vi "PAN_ProcCmd.vi"(0 "Translations":refnum<vi>, 1 "modpath":path, 4 "addid":refnum<vi>, 5 "Modules":refnum<vi>, 6 "cinfo":string, 7 "command in":string, 9 "exp time":dbl, 11 "shutdown":refnum<vi>, 12 "cmdQ":refnum<queue>, 13 "internal queue in":refnum<queue>, 14 "nodeID":string) -> (2 "init timeout":i32, 3 "DHE_DBSRef":T2, 8 "response":string, 10 "exp time out":dbl, 15 "shutdown":bool)   [LabVIEW 2016]
uses:
  Modules/DBSHAND/private/vis/DatabaseHand_RefNum.ctl
  PAN_actionsSTruct.ctl
  PAN_cmdStruct.ctl
panel:
  in  "action struct 2":T1
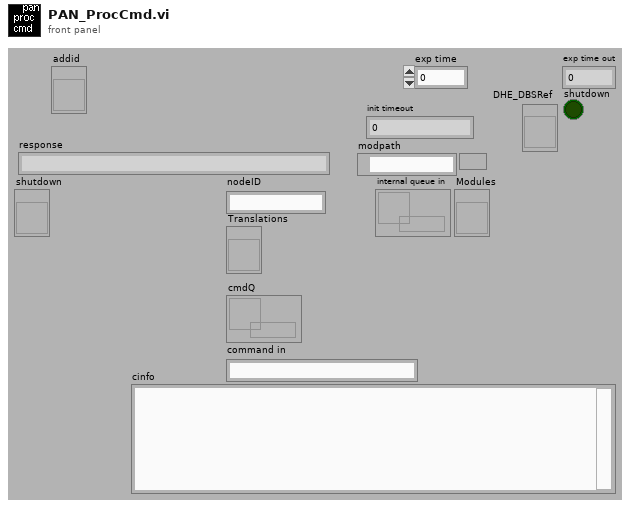
[diagram p1: front panel]
types:
  T1 = typedef "PAN_actionsSTruct.ctl" = cluster{"command":string, "timeout":u32}
  T2 = typedef "DatabaseHand_RefNum.ctl" = refnum<vi>
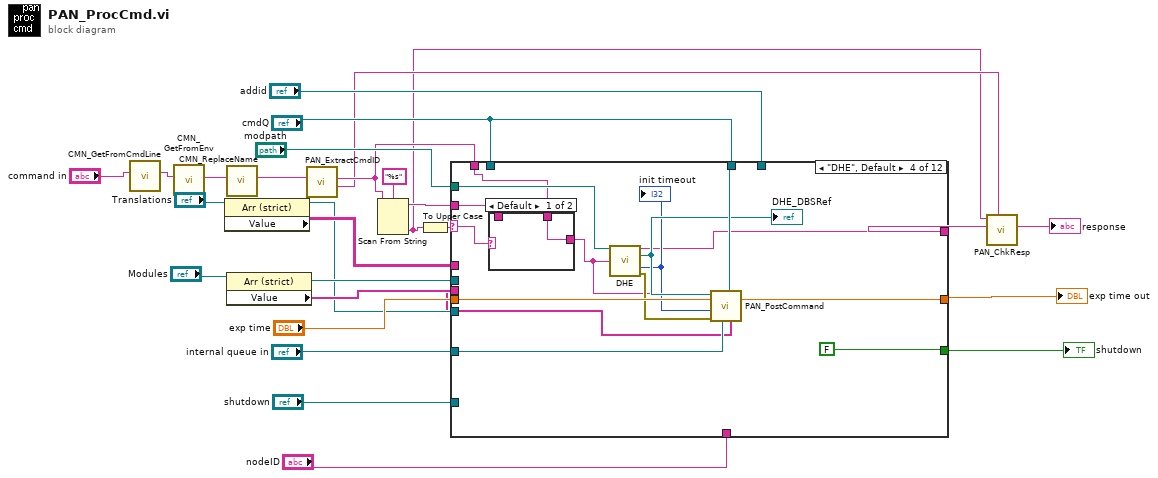
[diagram p0: block diagram]
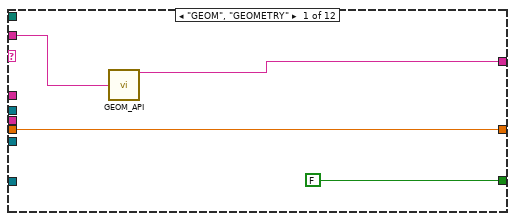
[diagram p2: hidden frame]
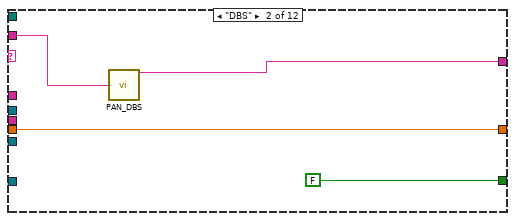
[diagram p3: hidden frame]
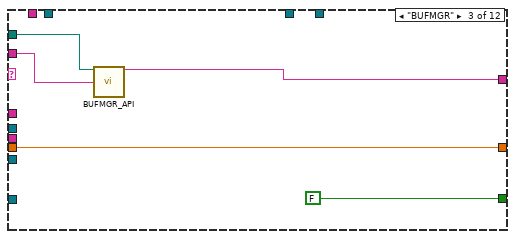
[diagram p4: hidden frame]
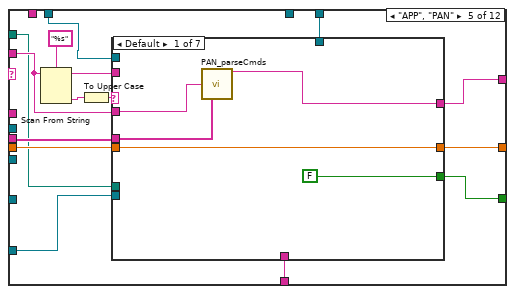
[diagram p6: hidden frame]
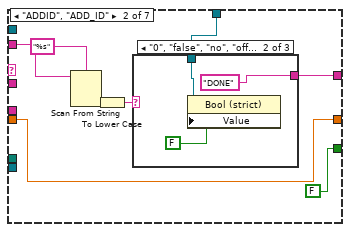
[diagram p7: hidden frame]
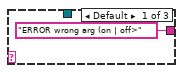
[diagram p8: hidden frame]
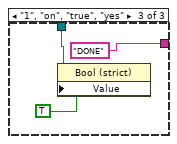
[diagram p9: hidden frame]
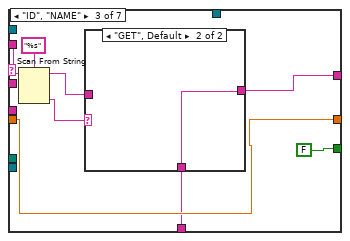
[diagram p10: hidden frame]
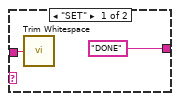
[diagram p11: hidden frame]
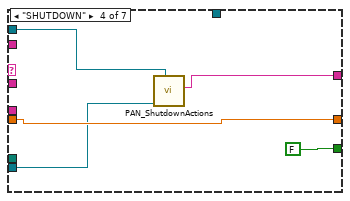
[diagram p12: hidden frame]
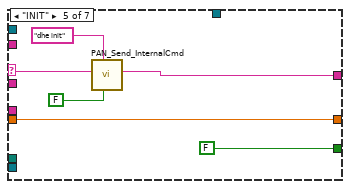
[diagram p13: hidden frame]
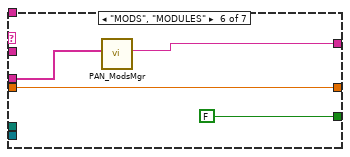
[diagram p14: hidden frame]
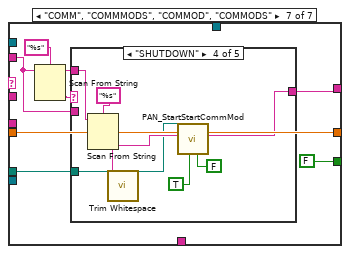
[diagram p15: hidden frame]
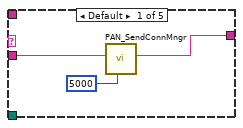
[diagram p16: hidden frame]
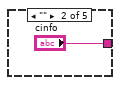
[diagram p17: hidden frame]
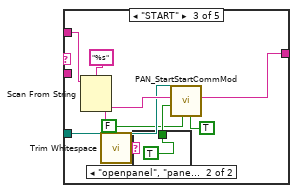
[diagram p18: hidden frame]
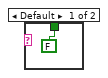
[diagram p19: hidden frame]
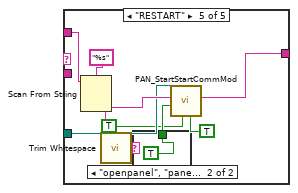
[diagram p20: hidden frame]
diagram:
  n1 = call "CMN_GetFromCmdLine.vi"("str in"="command in") -> ("str out"=w7:string)  [unwired: 10 out]
  n2 = call "CMN_GetFromEnv.vi"("str in"=w7) -> ("str out"=w5:string)  [unwired: 10 out]
  n3 = property class="Arr (strict)"(reference="Translations") -> (reference out=w12:refnum<vi>, "Value"=w13:string[][])  [unwired: 1 in, 1 out]
  n4 = call "CMN_ReplaceName.vi"("name in"=w5) -> ("name out"=w4:string)  [unwired: 1 in, 9 out]
  n5 = property class="Arr (strict)"(reference="Modules") -> (reference out=w15:refnum<vi>, "Value"=w16:string[])  [unwired: 1 in, 1 out]
  n6 = call "PAN_ExtractCmdID.vi"("command in"=w4) -> ("cmdID"=w2:string, "cmd out"=w3:string)  [unwired: 9 out]
  n7 = Scan From String(format string="%s", input string=w3) -> (remaining string=w25:string, output 1=w1:string)  [unwired: 2 in, 3 out]
  n8 = To Upper Case(1:w1) -> (0:w26:string)
  n9 = case shown="\"DHE\", Default" w26 {
    selector: w26 -> [_ _ _ w44 _ _ _ _ _ _ _ _]
    tunnel: w3 -> [_ _ _ w41 _ _ _ _ _ _ _ _]
    tunnel: [w31 w35 w40 w46 w68 w166 w171 w181 "DONE" ("ImmedReplyString") "DONE" ("ImmedReplyString") w211 "" ("ImmedReplyString")] -> w23
    tunnel: w25 -> [w29 w33 w38 w47 w63 w164 w169 w173 w195 _ _ _]
    tunnel: "exp time" -> [w30 w34 w39 w55 w65 w167 w172 w182 _ _ w212 _]
    tunnel: [w30 w34 w39 w54 w64 w167 w172 w182 0.0 ("exp time") 0.0 ("exp time") w212 0.0 ("exp time")] -> w24
    tunnel: "internal queue in" -> [_ _ _ w53 _ _ _ _ w198 _ _ _]
    tunnel: "cmdQ" -> [_ _ _ _ w67 _ _ _ _ w206 _ _]
    tunnel: "cmdQ" -> [_ _ _ w52 _ _ _ _ _ _ w210 _]
    tunnel: "modpath" -> [_ _ w37 w45 w58 _ _ w177 _ _ _ _]
    tunnel: w16 -> [_ _ _ w48 w66 _ _ w179 _ w203 _ _]
    tunnel: w13 -> [_ _ _ _ _ _ _ w180 _ _ _ _]
    tunnel: w15 -> [_ _ _ _ _ _ _ w176 _ _ _ _]
    tunnel: w12 -> [_ _ _ _ _ _ _ w175 _ _ _ _]
    tunnel: [FALSE FALSE FALSE FALSE w62 FALSE FALSE FALSE FALSE FALSE FALSE TRUE] -> w11
    tunnel: "nodeID" -> [_ _ _ _ w61 _ _ _ _ _ _ _]
    tunnel: "addid" -> [_ _ _ _ w60 _ _ _ _ _ _ _]
    tunnel: "shutdown" -> [_ _ _ _ w59 _ _ _ _ _ w209 _]
    frame "GEOM", "GEOMETRY" {
      n10 = call "GEOM_API.vi"("Cmd"=w29) -> ("ImmedReplyString"=w31:string)  [unwired: 1 in, 13 out]
    }
    frame "DBS" {
      n11 = call "PAN_DBS.vi"("Cmd"=w33) -> ("ImmedReplyString"=w35:string)  [unwired: 1 in, 13 out]
    }
    frame "BUFMGR" {
      n12 = call "BUFMGR_API.vi"("modpath"=w37, "Cmd"=w38) -> ("ImmedReplyString"=w40:string)  [unwired: 1 in, 12 out]
    }
    frame "DHE", Default {
      n13 = case shown="Default" w44 {
        tunnel: w41 -> [w56 _]
        tunnel: w47 -> [_ w57]
        tunnel: [w56 w57] -> w42
        frame Default {
        }
        frame "DHE" {
        }
      }
      n14 = call "DHE.vi"("modpath"=w45, "Cmd"=w42) -> ("ImmedReplyString"=w46:string, "DHE_DBSRef"=w51:T2, "TimeOut out"=w49:i32, "error out"=w50:errorcluster)  [unwired: 1 in, 9 out]
      "DHE_DBSRef" <- w51
      "init timeout" <- w49
      n15 = call "PAN_PostCommand.vi"("Modules"=w48, "cmdQ"=w52, "queue out"=w53, "command"=w42, "error in (no error)"=w50, "timeout"=w49, "orig exptime"=w55, "DHE_DBSRef"=w51) -> ("exp time"=w54:dbl)  [unwired: 3 out]
    }
    frame "APP", "PAN" {
      n16 = Scan From String(format string="%s", input string=w63) -> (remaining string=w69:string, output 1=w71:string)  [unwired: 2 in, 3 out]
      n17 = To Upper Case(1:w71) -> (0:w70:string)
      n18 = case shown="Default" w70 {
        selector: w70 -> [_ _ _ _ w112 _ _]
        tunnel: w69 -> [_ w85 w97 _ _ _ w121]
        tunnel: [w75 w78 w99 w106 w110 w117 w124] -> w68
        tunnel: [FALSE FALSE FALSE FALSE FALSE FALSE FALSE] -> w62
        tunnel: w67 -> [_ _ _ w105 _ _ _]
        tunnel: w66 -> [w73 _ _ _ _ w118 _]
        tunnel: w65 -> [w76 w80 w98 w107 w113 w116 w125]
        tunnel: [w76 w80 w98 w107 w113 w116 w125] -> w64
        tunnel: w63 -> [w74 _ _ _ _ _ _]
        tunnel: w61 -> [_ _ w93 _ _ _ _]
        tunnel: w60 -> [_ w79 _ _ _ _ _]
        tunnel: w59 -> [_ _ _ w104 _ _ _]
        tunnel: w58 -> [_ _ _ _ _ _ w119]
        frame Default {
          n19 = call "PAN_parseCmds.vi"("Cmd Option"=w74, "Modules"=w73) -> ("ImmedReplyString"=w75:string)  [unwired: 1 in, 12 out]
        }
        frame "ADDID", "ADD_ID" {
          n20 = Scan From String(format string="%s", input string=w85) -> (output 1=w82:string)  [unwired: 2 in, 4 out]
          n21 = To Lower Case(string=w82) -> (all lower case string=w81:string)
          n22 = case shown="\"0\", \"false\", \"no\", \"off\"" w81 {
            tunnel: w79 -> [_ w89 w92]
            tunnel: ["ERROR wrong arg (on | off>" ("response") "DONE" ("response") "DONE" ("response")] -> w78
            frame Default {
            }
            frame "0", "false", "no", "off" {
              n23 = property class="Bool (strict)"(reference=w89, "Value"=FALSE) -> ()  [unwired: 1 in, 2 out]
            }
            frame "1", "on", "true", "yes" {
              n24 = property class="Bool (strict)"(reference=w92, "Value"=TRUE) -> ()  [unwired: 1 in, 2 out]
            }
          }
        }
        frame "ID", "NAME" {
          n25 = Scan From String(format string="%s", input string=w97) -> (remaining string=w94:string, output 1=w95:string)  [unwired: 2 in, 3 out]
          n26 = case shown="\"GET\", Default" w95 {
            tunnel: ["DONE" ("ID") w103] -> w99
            tunnel: w94 -> [w101 _]
            tunnel: w93 -> [_ w103]
            frame "SET" {
              n27 = call <vilib>:"Trim Whitespace.vi"("string"=w101) -> ()  [unwired: 1 in, 1 out]
            }
            frame "GET", Default {
            }
          }
        }
        frame "SHUTDOWN" {
          n28 = call "PAN_ShutdownActions.vi"("cmdQ"=w105, "shutdownscr ref"=w104) -> ("response"=w106:string)  [unwired: 9 out]
        }
        frame "INIT" {
          n29 = call "PAN_Send_InternalCmd.vi"("wait response"=FALSE, "taskID"="dhe init", "command"=w112) -> ("response"=w110:string)  [unwired: 2 in, 6 out]
        }
        frame "MODS", "MODULES" {
          n30 = call "PAN_ModsMgr.vi"("Modules"=w118) -> ("response"=w117:string)  [unwired: 10 out]
        }
        frame "COMM", "COMMMODS", "COMMOD", "COMMODS" {
          n31 = Scan From String(format string="%s", input string=w121) -> (remaining string=w120:string, output 1=w122:string)  [unwired: 2 in, 3 out]
          n32 = case shown="\"SHUTDOWN\"" w122 {
            tunnel: [w127 "cinfo" w132 w144 w152] -> w124
            tunnel: w121 -> [w129 _ _ _ _]
            tunnel: w120 -> [_ _ w140 w150 w160]
            tunnel: w119 -> [_ _ w137 w147 w157]
            frame Default {
              n33 = call "PAN_SendConnMngr.vi"("timeout in ms (-1)"=5000, "command"=w129) -> ("resp"=w127:string)  [unwired: 1 in, 8 out]
            }
            frame "" {
            }
            frame "START" {
              n34 = Scan From String(format string="%s", input string=w140) -> (remaining string=w136:string, output 1=w138:string)  [unwired: 2 in, 3 out]
              n35 = call <vilib>:"Trim Whitespace.vi"("string"=w136) -> ("trimmed string"=w135:string)  [unwired: 1 in]
              n36 = case shown="\"openpanel\", \"panel\"" w135 {
                tunnel: [FALSE ("Front Panel Window:Open") TRUE ("Front Panel Window:Open")] -> w134
                frame Default {
                }
                frame "openpanel", "panel" {
                }
              }
              n37 = call "PAN_StartStartCommMod.vi"("start"=TRUE, "running"=FALSE, "ModPath"=w137, "openpanel"=w134, "commod"=w138) -> ("response"=w132:string)  [unwired: 1 in, 5 out]
            }
            frame "SHUTDOWN" {
              n38 = Scan From String(format string="%s", input string=w150) -> (remaining string=w146:string, output 1=w148:string)  [unwired: 2 in, 3 out]
              n39 = call <vilib>:"Trim Whitespace.vi"("string"=w146) -> ()  [unwired: 1 in, 1 out]
              n40 = call "PAN_StartStartCommMod.vi"("start"=FALSE, "running"=TRUE, "ModPath"=w147, "commod"=w148) -> ("response"=w144:string)  [unwired: 2 in, 5 out]
            }
            frame "RESTART" {
              n41 = Scan From String(format string="%s", input string=w160) -> (remaining string=w156:string, output 1=w158:string)  [unwired: 2 in, 3 out]
              n42 = call <vilib>:"Trim Whitespace.vi"("string"=w156) -> ("trimmed string"=w155:string)  [unwired: 1 in]
              n43 = case shown="\"openpanel\", \"panel\"" w155 {
                tunnel: [FALSE ("Front Panel Window:Open") TRUE ("Front Panel Window:Open")] -> w154
                frame Default {
                }
                frame "openpanel", "panel" {
                }
              }
              n44 = call "PAN_StartStartCommMod.vi"("start"=TRUE, "running"=TRUE, "ModPath"=w157, "openpanel"=w154, "commod"=w158) -> ("response"=w152:string)  [unwired: 1 in, 5 out]
            }
          }
        }
      }
    }
    frame "APPMACRO" {
      n45 = call "PAN_MacroCmd.vi"("timeout in ms (-1)"=-1, "Command"=w164) -> ("response"=w166:string)  [unwired: 1 in, 8 out]
    }
    frame "APPMACRONORESP" {
      n46 = call "PAN_MacroCmd.vi"("timeout in ms (-1)"=1, "Command"=w169) -> ("response"=w171:string)  [unwired: 1 in, 8 out]
    }
    frame "MOD" {
      n47 = call "PAN_ModCaller.vi"("CmdStringIn"=w173, "modpath"=w177) -> ("ImmedReplyString"=w181:string, "new mod"=w178:bool)  [unwired: 1 in, 11 out]
      n48 = case shown="True" w178 {
        tunnel: w180 -> [_ w190]
        tunnel: w179 -> [_ w189]
        tunnel: w173 -> [_ w188]
        tunnel: w177 -> [_ w187]
        tunnel: w176 -> [_ w186]
        tunnel: w175 -> [_ w184]
        frame False {
        }
        frame True {
          n49 = call "PAN_AddModule.vi"("Mods in"=w189, "Translations In"=w190, "modpath"=w187, "module name"=w188) -> ("Mods Out"=w185:string[], "Translations out"=w183:string[][])  [unwired: 6 out]
          n50 = property class="Arr (strict)"(reference=w186, "Value"=w185) -> ()  [unwired: 1 in, 2 out]
          n51 = property class="Arr (strict)"(reference=w184, "Value"=w183) -> ()  [unwired: 1 in, 2 out]
        }
      }
    }
    frame "BOOT" {
      n52 = Scan From String(format string="%d", input string=w195) -> (output 1=w193:i32)  [unwired: 2 in, 4 out]
      n53 = Bundle By Name(cluster="action struct 2", "command"="INIT", "timeout"=w193) -> (w200:T1)
      n54 = call "PAN_VAR_Status.vi"("action"=enum16{"read", "write", "set_ref"}."write", "status in"="sending init command  ...") -> ()  [unwired: 2 in, 8 out]
      n55 = Enqueue Element(queue=w198, element=w200) -> ()  [unwired: 1 in, 4 out]
    }
    frame "_SHUTDOWN_" {
      n56 = call "PAN_Shutdown.vi"("cmdQ"=w206, "Modules"=w203) -> ()  [unwired: 10 out]
      n57 = call "PAN_parseCmds.vi"("Cmd Option"="SHUTDOWN") -> ()  [unwired: 2 in, 13 out]
    }
    frame "SHUTDOWN" {
      n58 = call "PAN_ShutdownActions.vi"("cmdQ"=w210, "shutdownscr ref"=w209) -> ("response"=w211:string)  [unwired: 9 out]
    }
    frame "BYE" {
    }
  }
  "exp time out" <- w24
  "shutdown" <- w11
  n59 = call "PAN_ChkResp.vi"("cmdID  in"=w2, "resp in"=w23, "source"=w1) -> ("resp out"=→"response":string)  [unwired: 8 out]
